vi "CountLicks.vi"(5 "StageMoving?":bool, 6 "Start time":u32, 7 "LickPerMinIn":i32[][](array[numeric]), 8 "NLicks In":i32[](array[numeric]), 9 "Previous Lick State":dbl, 10 "Current Lick State":dbl) -> (0 "LickPerMinOut":i32[][](array[numeric]), 1 "NLicksOut":i32[](array[numeric]), 2 "NewVal?":bool, 3 "Current Lick State Out":dbl)   [LabVIEW 2013]
panel:
  out "floor(x/y)":u32
  out "size(s)":i32[](array[numeric])
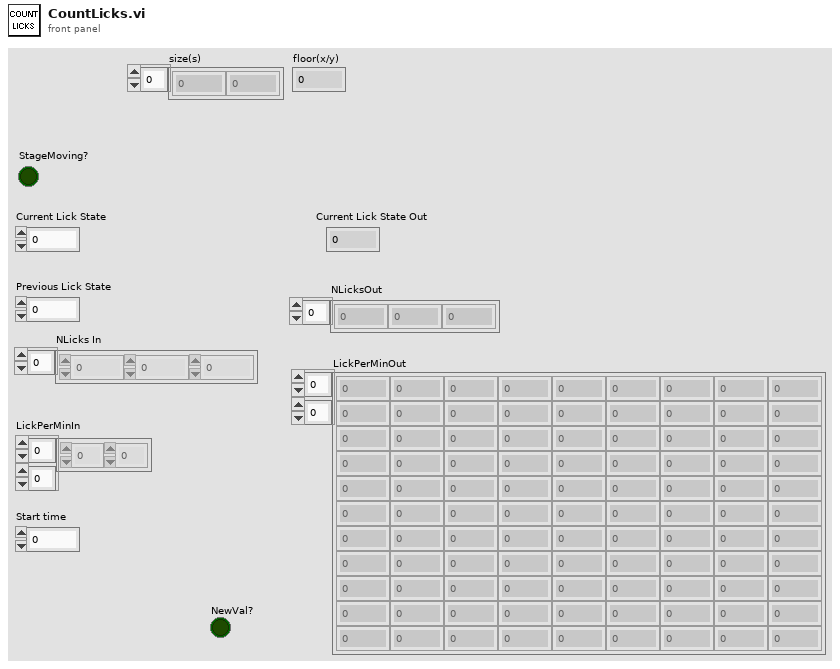
[diagram p1: front panel]
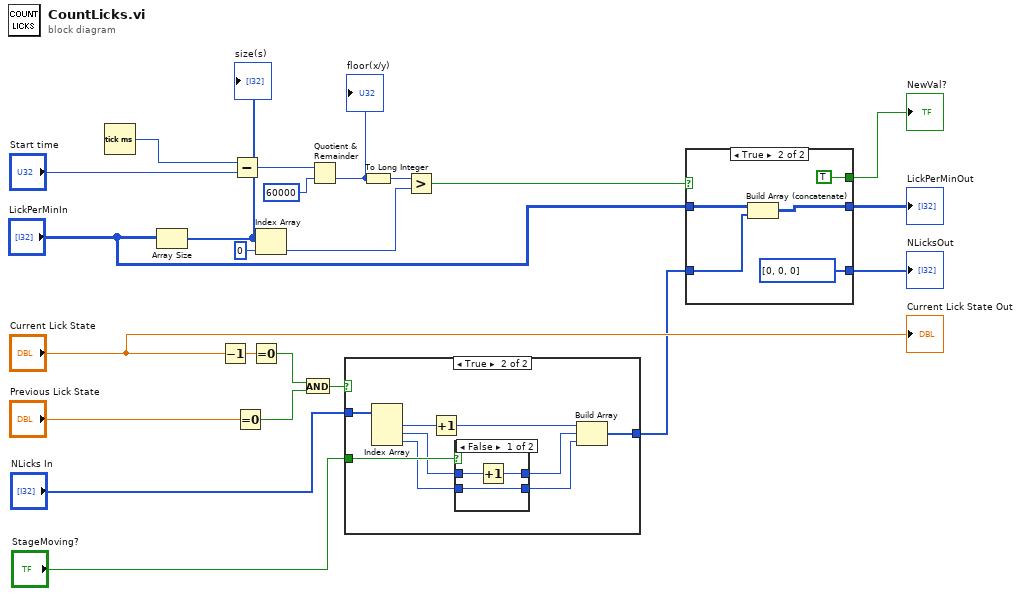
[diagram p0: block diagram]
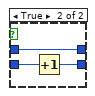
[diagram p3: hidden frame]
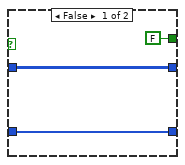
[diagram p4: hidden frame]
diagram:
  n1 = Tick Count (ms)() -> (millisecond timer value=w21:u32)
  n2 = Array Size(array="LickPerMinIn") -> (size(s)=w8:i32[])
  "size(s)" <- w8
  n3 = Decrement(x="Current Lick State") -> (x-1=w11:dbl)
  n4 = Subtract(x=w21, y="Start time") -> (x-y=w19:u32)
  n5 = Equal To 0?(x="Previous Lick State") -> (x = 0?=w14:bool)
  n6 = Equal To 0?(x=w11) -> (x = 0?=w13:bool)
  n7 = Index Array(array=w8, index=0) -> (element=w6:i32)
  n8 = And(x=w13, y=w14) -> (x .and. y?=w12:bool)
  n9 = Quotient & Remainder(x=w19, y=u32 60000) -> (floor(x/y)=w17:u32)  [unwired: 1 out]
  "floor(x/y)" <- w17
  n10 = case shown="True" w12 {
    tunnel: "NLicks In" -> [w24 w33]
    tunnel: [w24 w25] -> w10
    tunnel: "StageMoving?" -> [_ w30]
    frame False {
    }
    frame True {
      n11 = Index Array(array=w33) -> (element #1=w31:i32, element #2=w29:i32, element #3=w28:i32)  [unwired: 3 in]
      n12 = Increment(x=w31) -> (x+1=w32:i32)
      n13 = case shown="False" w30 {
        tunnel: w29 -> [w36 w37]
        tunnel: w28 -> [w34 w39]
        tunnel: [w35 w37] -> w27
        tunnel: [w34 w38] -> w26
        frame False {
          n14 = Increment(x=w36) -> (x+1=w35:i32)
        }
        frame True {
          n15 = Increment(x=w39) -> (x+1=w38:i32)
        }
      }
      n16 = Build Array(w32, w27, w26) -> (w25:i32[])
    }
  }
  n17 = To Long Integer(number=w17) -> (32bit integer=w16:i32)
  n18 = Greater?(x=w16, y=w6) -> (0:w15:bool)
  n19 = case shown="True" w15 {
    tunnel: w10 -> [w42 w46]
    tunnel: "LickPerMinIn" -> [w41 w47]
    tunnel: [w41 w45] -> w5
    tunnel: [w42 i32[] [0, 0, 0]] -> w4
    tunnel: [FALSE TRUE] -> w1
    frame False {
    }
    frame True {
      n20 = Build Array (concatenate)(w47, w46) -> (w45:i32[][])
    }
  }
  "LickPerMinOut" <- w5
  "NewVal?" <- w1
  "NLicksOut" <- w4
  "Current Lick State Out" <- "Current Lick State"
